vi "splash.vi"() -> ()   [LabVIEW 2020]
panel:
  out "logo":picture
  # "Copyright 2022. All rights reserved"
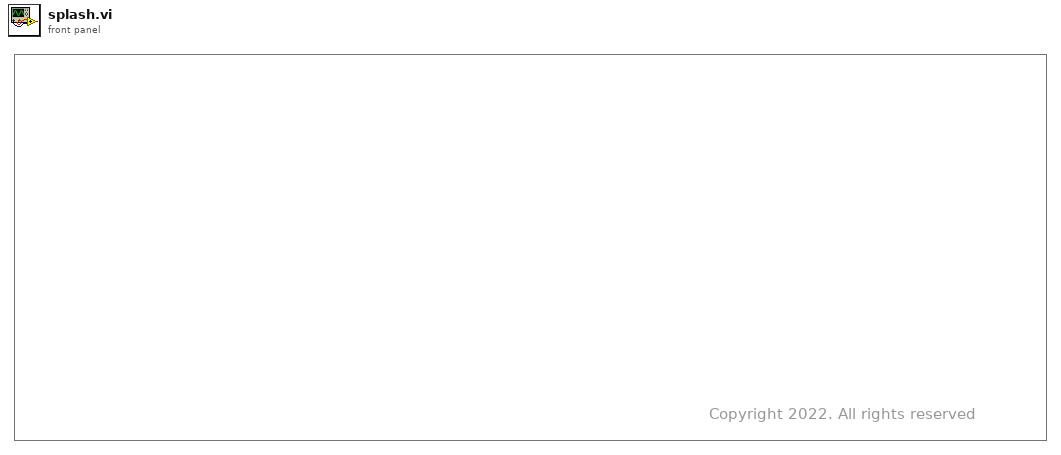
[diagram p1: front panel]
types:
  T1 = typedef "imagedata.ctl" = cluster{"image type":i32, "image depth":i32, "image":u8[], "mask":u8[], "colors":u32[], "Rectangle":cluster{"left":i16, "top":i16, "right":i16, "bottom":i16}}
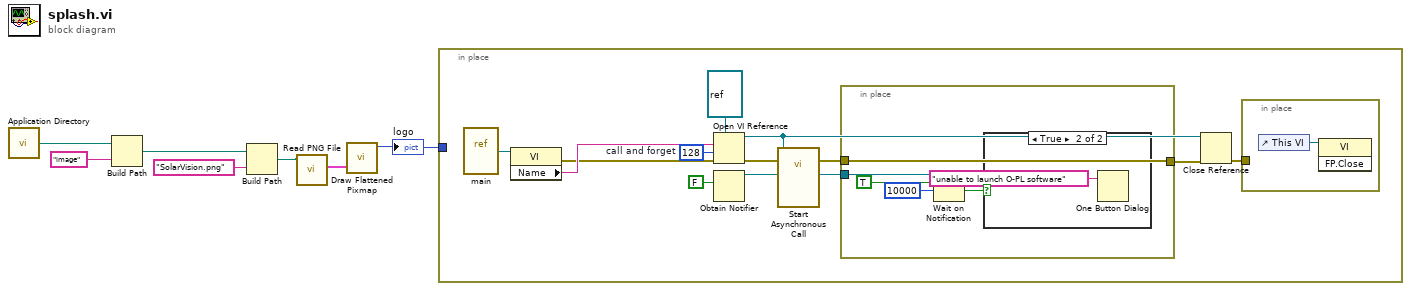
[diagram p0: block diagram]
diagram:
  n1 = call <vilib>:"Application Directory.vi"() -> ("Application Directory"=w3:path)
  n2 = Build Path(base path=w3, name or relative path="image" ("VI Name")) -> (appended path=w4:path)
  n3 = Build Path(base path=w4, name or relative path="SolarVision.png" ("VI Name")) -> (appended path=w6:path)
  n4 = call <vilib>:"Read PNG File.vi"("path to PNG file"=w6) -> ("image data"=w7:T1)  [unwired: 8 in, 2 out]
  n5 = call <vilib>:"Draw Flattened Pixmap.vi"("image data"=w7) -> ("new picture"=w1:picture)  [unwired: 8 in]
  "logo" <- w1
  n6 = in-place {
    in-place-border: w1 -> [_]
    w19 = 128  # call and forget
    n7 = vi-ref "main.vi"() -> (w17:refnum<vi>)
    n8 = property class="VI"(reference=w17) -> (error out=w14:errorcluster, "Name"=w16:string)  [unwired: 1 in, 1 out]
    n9 = Open VI Reference(type specifier VI Refnum (for type only)=refnum<vi> refnum, vi path=w16, options=w19, error in (no error)=w14) -> (vi reference=w11:refnum<vi>, error out=w15:errorcluster)  [unwired: 2 in]
    n10 = Obtain Notifier(notification data type=FALSE) -> (notifier out=w12:refnum<notifier>)  [unwired: 3 in, 2 out]
    n11 = call-by-ref "Start Asynchronous Call"(reference=w11, error in=w15, "launched"=w12) -> (error out=w10:errorcluster)  [unwired: 11 in, 1 out]
    n12 = in-place {
      in-place-border: w12 -> [w24]
      in-place-border: [w20] -> w9
      in-place-border: w10 -> [w20]
      n13 = Wait on Notification(notifier=w24, ignore previous (F)=TRUE, timeout in ms (-1)=10000) -> (timed out?=w21:bool)  [unwired: 1 in, 3 out]
      n14 = case shown="True" w21 {
        frame False {
        }
        frame True {
          n15 = One Button Dialog(message="unable to launch O-PL software") -> ()  [unwired: 1 in, 1 out]
        }
      }
    }
    n16 = Close Reference(reference=w11, error in (no error)=w9) -> (error out=w8:errorcluster)
    n17 = in-place {
      in-place-border: w8 -> [_]
      n18 = control-ref of="This VI"() -> (w26:refnum<vi>)
      n19 = invoke class="VI" method="FP.Close"(reference=w26) -> ()  [unwired: 2 in, 3 out]
    }
  }
